vi "mie-demo-Lior.vi"(0 "refractive index, real":sgl=1.3 step=0.01 format="%.2f", 1 "Number of Measurements":i32, 2 "refractive index, imaginary":sgl=0.1 step=0.01 format="%.2f", 3 "max size parameter alpha\n(alpha = 2Pi*r/lambda)":sgl=1.0 step=0.01 format="%.2f", 4 "Number of particle sizes of measurements":i32, 5 "Uncertainty (sigma) in percentages from the mean":i32) -> (6 "Extinction Graph":cluster{"Ramp Pattern":dbl[], dbl[]}[](graph), 7 "Absorption Graph":cluster{"Y":dbl[], "Y":dbl[]}[](graph), 8 "X Mean std error Expected extinction":T1)   [LabVIEW 2011]
uses:
  <vilib>/Analysis/1siggen.llb/Ramp Pattern by Samples.vi
  <vilib>/gmath/statdist.llb/Normal Random.vi
  mie2.dll
  <vilib>/Analysis/NI_AALBase.lvlib
  <vilib>/gmath/NI_Gmath.lvlib
panel:
  out "totalscatter 2":sgl
  out "backscatter 2":sgl
  out "<cos(theta)> 3":sgl
  out "extinction 2":sgl
  out "extinction":sgl
  in  "Number of particle sizes for expected values":i32
  out "<cos(theta)> 2":sgl
  out "backscatter":sgl
  out "totalscatter":sgl
  in  "angles (will compute\n2*angles-1 points from\n0...180 degrees)":u32=181
  # "Mie scattering demo program, August 2005, by Martin Fierz (martin@fierz.ch)\n\nThis VI demonstrates the usage of mie2.dll; a dynamic-link-library which you can call in your LabView program.\nThe demo lets you select the refractive index of a sphere, and the size parameter and computes total scattering,\ntotal extinction and angular distribution of the scattered light for p-, s- and unpolarized light.\nMie2.dll uses the Bohren-Huffman Mie code."
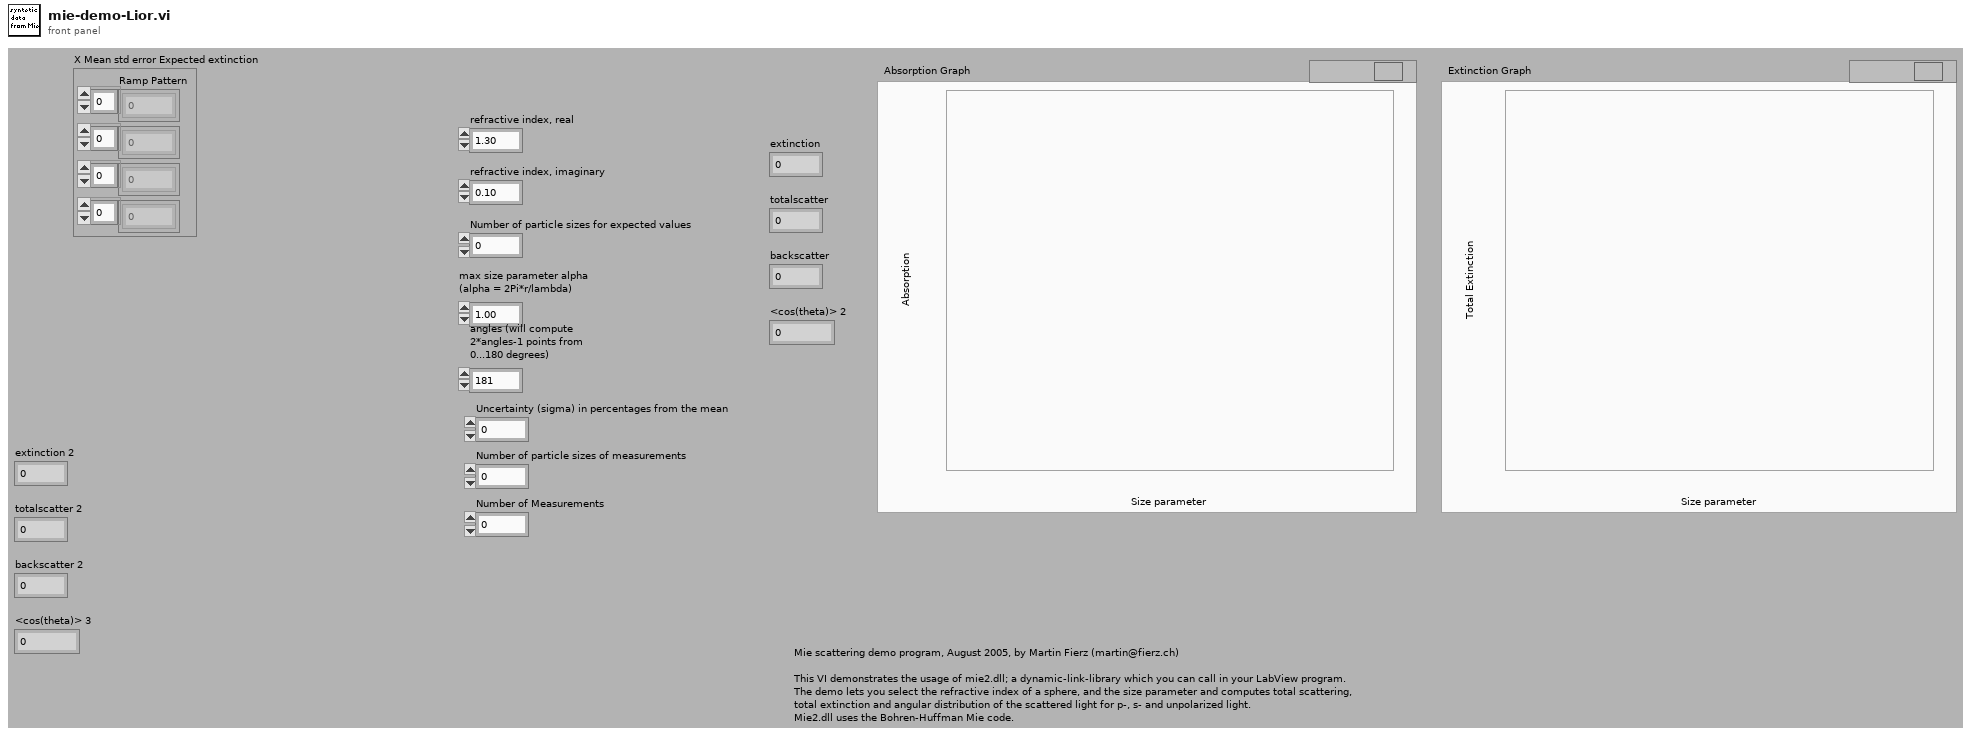
[diagram p1: front panel]
types:
  T1 = cluster{"Ramp Pattern":dbl[], dbl[], dbl[], sgl[]}
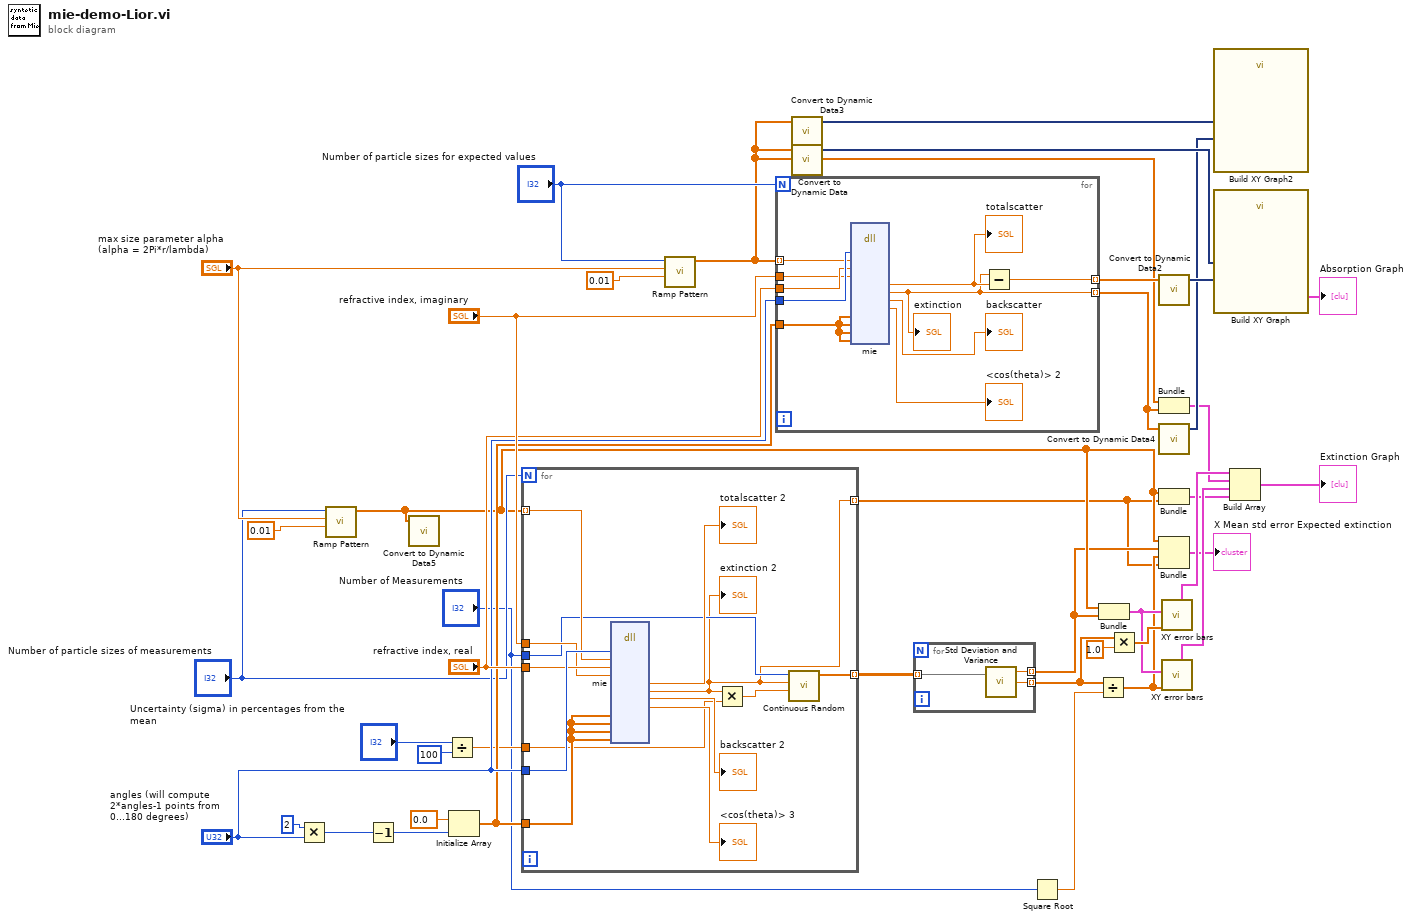
[diagram p0: block diagram]
diagram:
  n1 = Multiply(x=u32 2, y="angles (will compute\n2*angles-1 points from\n0...180 degrees)") -> (x*y=w40:u32)
  n2 = call-poly <vilib>:"Ramp Pattern.vi"("start"=0.01, "end"="max size parameter alpha\n(alpha = 2Pi*r/lambda)", "samples"="Number of particle sizes of measurements") -> ("Ramp Pattern"=w7:dbl[])  [unwired: 7 in, 1 out]
  n3 = Decrement(x=w40) -> (x-1=w38:u32)
  n4 = call "Convert to Dynamic Data5"("Array"=w7) -> ()  [unwired: 3 in, 1 out]
  n5 = Divide(x="Uncertainty (sigma) in percentages from the mean", y=100) -> (x/y=w21:dbl)
  n6 = Initialize Array(sgl 0.0, w38) -> (w26:sgl[])
  n7 = for {
    N: "Number of particle sizes of measurements" -> [_]
    tunnel: w26 -> [w52]
    tunnel: "angles (will compute\n2*angles-1 points from\n0...180 degrees)" -> [w51]
    tunnel: "refractive index, real" -> [w50]
    tunnel: "refractive index, imaginary" -> [w49]
    tunnel: w7 -> [w48] mode=indexing
    tunnel: w21 -> [w46]
    tunnel: [w45] -> w20 mode=indexing
    tunnel: "Number of Measurements" -> [w44]
    tunnel: [w42] -> w1 mode=indexing
    n8 = dll-call lib="Z:/Dropbox/Lior Segev/Lior Segev Projects/BAES data analysis/mie2.dll" fn="mie"("angles"=w51, "x"=w48, "r"=w50, "i"=w49, "spol_real"=w52, "spol_imaginary"=w52, "ppol_real"=w52, "ppol_imaginary"=w52) -> ("totalscatter"=→"totalscatter 2":sgl, "extinction"=w42:sgl, "backscatter"=→"backscatter 2":sgl, "<cos(theta)>"=→"<cos(theta)> 3":sgl)  [unwired: 16 in, 2 out]
    "extinction 2" <- w42
    n9 = Multiply(x=w42, y=w46) -> (x*y=w43:dbl)
    n10 = call-poly <vilib>:"Continuous Random.vi"("std"=w43, "mean"=w42, "samples"=w44) -> ("normal random data"=w45:dbl[])  [unwired: 7 in, 1 out]
  }
  n11 = call-poly <vilib>:"Ramp Pattern.vi"("start"=0.01, "end"="max size parameter alpha\n(alpha = 2Pi*r/lambda)", "samples"="Number of particle sizes for expected values") -> ("Ramp Pattern"=w17:dbl[])  [unwired: 7 in, 1 out]
  n12 = for {
    N: "Number of particle sizes for expected values" -> [_]
    tunnel: w26 -> [w62]
    tunnel: "angles (will compute\n2*angles-1 points from\n0...180 degrees)" -> [w61]
    tunnel: "refractive index, real" -> [w60]
    tunnel: "refractive index, imaginary" -> [w59]
    tunnel: [w56] -> w35 mode=indexing
    tunnel: w17 -> [w58] mode=indexing
    tunnel: [w55] -> w3 mode=indexing
    n13 = dll-call lib="Z:/Dropbox/Lior Segev/Lior Segev Projects/BAES data analysis/mie2.dll" fn="mie"("angles"=w61, "x"=w58, "r"=w60, "i"=w59, "spol_real"=w62, "spol_imaginary"=w62, "ppol_real"=w62, "ppol_imaginary"=w62) -> ("totalscatter"=w57:sgl, "extinction"=w55:sgl, "backscatter"=→"backscatter":sgl, "<cos(theta)>"=→"<cos(theta)> 2":sgl)  [unwired: 16 in, 2 out]
    "totalscatter" <- w57
    "extinction" <- w55
    n14 = Subtract(x=w55, y=w57) -> (x-y=w56:sgl)
  }
  n15 = call "Convert to Dynamic Data3"("Array"=w17) -> ("Dynamic Data Type"=w31:dynamicdata)  [unwired: 3 in]
  n16 = call "Convert to Dynamic Data"("Array"=w17) -> ("Dynamic Data Type"=w36:dynamicdata)  [unwired: 3 in]
  n17 = for {
    tunnel: w20 -> [w67] mode=indexing
    tunnel: [w66] -> w6 mode=indexing
    tunnel: [w65] -> w12 mode=indexing
    n18 = call <vilib>:"Std Deviation and Variance.vi"("X"=w67) -> ("mean"=w66:dbl, "standard deviation"=w65:dbl)  [unwired: 1 in, 1 out]
  }
  n19 = Square Root(x="Number of Measurements") -> (sqrt(x)=w19:dbl)
  n20 = Divide(x=w12, y=w19) -> (x/y=w4:dbl[])
  n21 = Bundle("Ramp Pattern"=w7, w6) -> (w10:cluster{"Ramp Pattern":dbl[], dbl[]})  [unwired: 1 in]
  n22 = Multiply(x=w12, y=1.0) -> (x*y=w11:dbl[])
  n23 = call "Convert to Dynamic Data2"("Array"=w35) -> ("Dynamic Data Type"=w34:dynamicdata)  [unwired: 3 in]
  n24 = Bundle("Ramp Pattern"=w17, w3) -> (w15:cluster{"Ramp Pattern":dbl[], sgl[]})  [unwired: 1 in]
  n25 = call "Convert to Dynamic Data4"("Array"=w3) -> ("Dynamic Data Type"=w30:dynamicdata)  [unwired: 3 in]
  n26 = Bundle("Ramp Pattern"=w7, w1) -> (w8:cluster{"Ramp Pattern":dbl[], sgl[]})  [unwired: 1 in]
  n27 = Bundle("Ramp Pattern"=w7, w6, w4, w1) -> (→"X Mean std error Expected extinction":T1)  [unwired: 1 in]
  n28 = call "XY error bars.vi"("XY plot"=w10, "Yerror"=w11) -> ("Y error bars"=w16:cluster{dbl[], dbl[]})  [unwired: 6 in, 2 out]
  n29 = call "XY error bars.vi"("XY plot"=w10, "Yerror"=w4) -> ("Y error bars"=w9:cluster{dbl[], dbl[]})  [unwired: 6 in, 2 out]
  n30 = call "Build XY Graph2"("Y Input"=w30, "X Input"=w31) -> ()  [unwired: 3 in, 7 out]
  n31 = call "Build XY Graph"("Y Input"=w34, "X Input"=w36) -> ("XY Graph"=→"Absorption Graph":cluster{"Y":dbl[], "Y":dbl[]}[])  [unwired: 3 in, 6 out]
  n32 = Build Array(w16, w15, w9, w8) -> (→"Extinction Graph":cluster{"Ramp Pattern":dbl[], dbl[]}[])
